vi "ccc_Convert To Compatibility Conn ID.vi"(11 "new connection ID":T1) -> (3 "old connection ID":T7)   [LabVIEW 2010]
uses:
  ccc_ConnectionID.ctl
  <vilib>/NI/STM/compatibility/stm_TCP Connection Info.ctl
  <vilib>/NI/STM/compatibility/stm_MetaDataElement.ctl
  ccc_TagConfiguration.ctl
  <vilib>/NI/Current Value Table/Compatibility/_SubVIs/TypeDefs/cvt_Data Types.ctl
  ccc_TagDirection.ctl
  Connection ID.ctl
  <vilib>/NI/STM/TCP/TCP Connection Info.ctl
  <vilib>/NI/STM/SubVIs/MetaDataElement.ctl
  Tag Configuration.ctl
  <vilib>/NI/Current Value Table/Type Defs/Data Types.ctl
  Tag Direction.ctl
  <vilib>/NI/Current Value Table/Current Value Table.lvlib
  NI_CCC.lvlib
  <vilib>/NI/STM/NI STM.lvlib
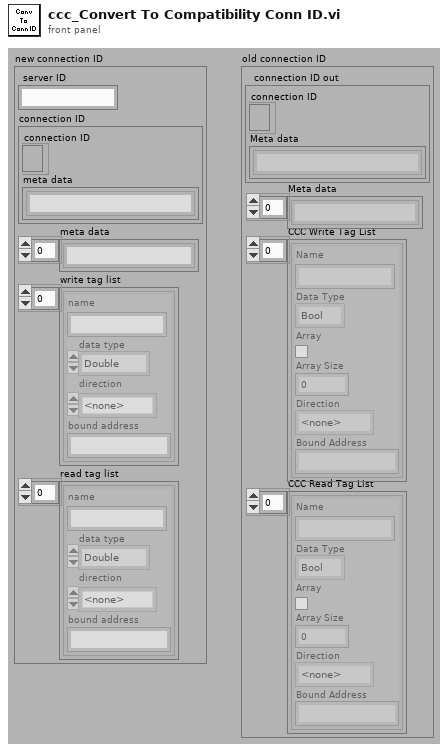
[diagram p1: front panel]
types:
  T1 = typedef "NI_CCC.lvlib/Connection ID.ctl" = cluster{"server ID":string, "connection ID":T2, "meta data":T3[], "write tag list":T4[], "read tag list":T4[]}
  T2 = typedef "NI STM.lvlib/TCP Connection Info.ctl" = cluster{"connection ID":refnum<k5>, "meta data":T3[]}
  T3 = typedef "NI STM.lvlib/MetaDataElement.ctl" = string
  T4 = typedef "NI_CCC.lvlib/Tag Configuration.ctl" = cluster{"name":string, "data type":T5, "direction":T6, "bound address":string}
  T5 = typedef "Current Value Table.lvlib/Data Types.ctl" = enum16{"Double", "Single", "I64", "I32", "I16", "I8", "U64", "U32", "U16", "U8", "String", "Boolean", "Array of U8", "Array of U16", "Array of U32", "Array of U64", "Array of I64", "Array of I32", "Array of I16", "Array of I8", "Array of Double", "Array of Single", "Array of Boolean", "Array of String"}
  T6 = typedef "NI_CCC.lvlib/Tag Direction.ctl" = enum32{"<none>", "Read", "Write"}
  T7 = typedef "ccc_ConnectionID.ctl" = cluster{"connection ID out":T8, "Meta data":T9[], "CCC Write Tag List":T10[], "CCC Read Tag List":T10[]}
  T8 = typedef "stm_TCP Connection Info.ctl" = cluster{"connection ID":refnum<k5>, "Meta data":T9[]}
  T9 = typedef "stm_MetaDataElement.ctl" = string
  T10 = typedef "ccc_TagConfiguration.ctl" = cluster{"Name":string, "Data Type":T11, "Array":bool, "Array Size":u32, "Direction":T12, "Bound Address":string}
  T11 = typedef "cvt_Data Types.ctl" = enum16{"Bool", "U8", "I32", "Double", "String", "Enum"}
  T12 = typedef "ccc_TagDirection.ctl" = enum32{"<none>", "Read", "Write"}
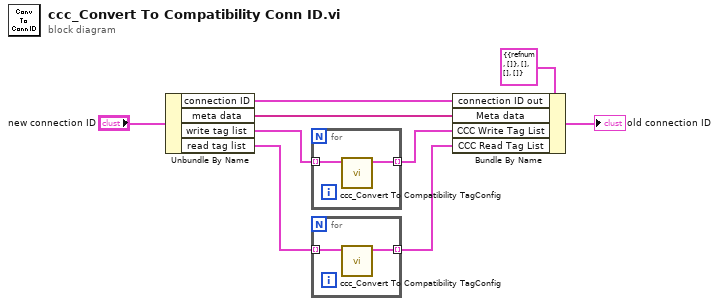
[diagram p0: block diagram]
diagram:
  n1 = Unbundle By Name("new connection ID") -> ("connection ID"=w9:T2, "meta data"=w8:T3[], "write tag list"=w7:T4[], "read tag list"=w2:T4[])
  n2 = for {
    tunnel: w7 -> [w11] mode=indexing
    tunnel: [w10] -> w6 mode=indexing
    n3 = call "ccc_Convert To Compatibility TagConfig.vi"("new tag"=w11) -> ("old tag"=w10:T10)  [unwired: 10 in]
  }
  n4 = for {
    tunnel: w2 -> [w13] mode=indexing
    tunnel: [w12] -> w1 mode=indexing
    n5 = call "ccc_Convert To Compatibility TagConfig.vi"("new tag"=w13) -> ("old tag"=w12:T10)  [unwired: 10 in]
  }
  n6 = Bundle By Name(cluster=T7 {"connection ID out"={"connection ID"=refnum, "Meta data"=[]}, "Meta data"=[], "CCC Write Tag List"=[], "CCC Read Tag List"=[]} ("old connection ID"), "connection ID out"=w9, "Meta data"=w8, "CCC Write Tag List"=w6, "CCC Read Tag List"=w1) -> (→"old connection ID":T7)
